vi "Throw -8716 error.vi"(8 "error in (no error)":errorcluster, 9 "dir speed name":string, 10 "tooth source name":string, 11 "error":bool) -> (0 "error out":errorcluster)   [LabVIEW 2013, in "Engine Simulation Toolkit System Explorer.lvlib"]
uses:
  Engine Simulation Toolkit System Explorer.lvlib
  <vilib>/Utility/error.llb/Error Cluster From Error Code.vi
  <vilib>/ErrorRing/Error Ring.xnode
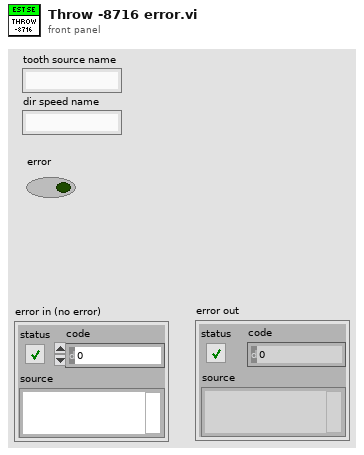
[diagram p1: front panel]
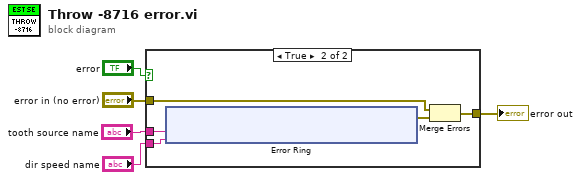
[diagram p0: block diagram]
diagram:
  n1 = case shown="True" "error" {
    tunnel: "error in (no error)" -> [w6 w11]
    tunnel: "tooth source name" -> [_ w9]
    tunnel: [w6 w8] -> w5
    tunnel: "dir speed name" -> [_ w7]
    frame False {
    }
    frame True {
      n2 = xnode "Error Ring"("parameter 0"=w9, "parameter 1"=w7) -> ("error out"=w10:errorcluster)
      n3 = Merge Errors(w11, w10) -> (w8:errorcluster)
    }
  }
  "error out" <- w5
